vi "Order Controls.vi"(10 "TermBnds[]":T1[](array[typedef]), 11 "Controls in":refnum<vi>[](array[refnum])) -> (1 "sorted array":cluster{"Rectangle":T1, refnum<vi>}[](array[cluster]), 2 "Control locations":T1[](array[typedef]), 3 "Controls out":refnum<vi>[](array[refnum]))   [LabVIEW 2014]
uses:
  <vilib>/Utility/miscctls.llb/LVRectTypeDef.ctl
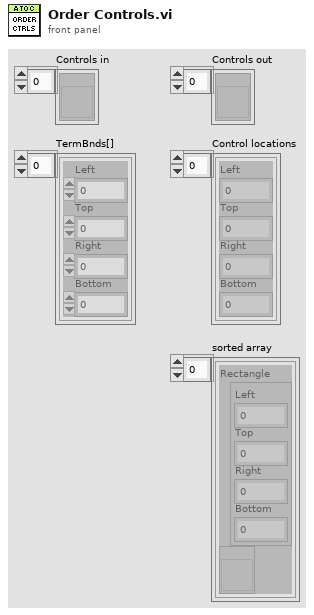
[diagram p1: front panel]
types:
  T1 = typedef "LVRectTypeDef.ctl" = cluster{"Left":i16, "Top":i16, "Right":i16, "Bottom":i16}
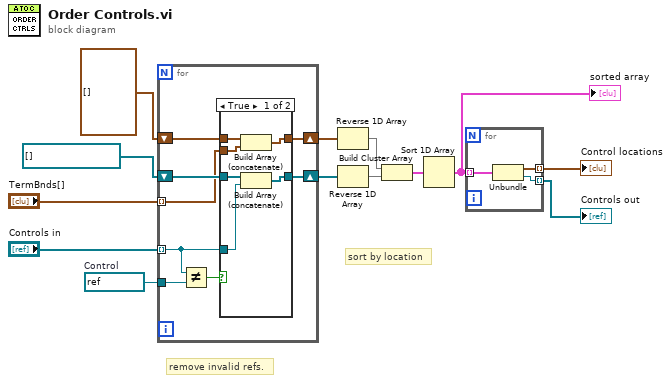
[diagram p0: block diagram]
diagram:
  w13 = refnum<vi> refnum  # Control
  # "sort by location"
  # "remove invalid refs."
  n1 = for {
    tunnel: w13 -> [w17]
    shift-right: [w20] -> w7
    shift-left: refnum<vi>[] [] ("Controls in") -> [w21]
    shift-right: [w18] -> w8
    shift-left: T1[] [] ("TermBnds[]") -> [w19]
    tunnel: "Controls in" -> [w15] mode=indexing
    tunnel: "TermBnds[]" -> [w14] mode=indexing
    n2 = Not Equal?(x=w15, y=w17) -> (x != y?=w16:bool)
    n3 = case shown="True" w16 {
      tunnel: w21 -> [w27 w29]
      tunnel: [w25 w29] -> w20
      tunnel: w19 -> [w26 w28]
      tunnel: [w24 w28] -> w18
      tunnel: w15 -> [w23 _]
      tunnel: w14 -> [w22 _]
      frame True {
        n4 = Build Array (concatenate)(w26, w22) -> (w24:T1[])
        n5 = Build Array (concatenate)(w27, w23) -> (w25:refnum<vi>[])
      }
      frame False {
      }
    }
  }
  n6 = Reverse 1D Array(array=w8) -> (reversed array=w4:T1[])
  n7 = Reverse 1D Array(array=w7) -> (reversed array=w3:refnum<vi>[])
  n8 = Build Cluster Array(w4, w3) -> (w2:cluster{"Rectangle":T1, refnum<vi>}[])
  n9 = Sort 1D Array(array=w2) -> (sorted array=w1:cluster{"Rectangle":T1, refnum<vi>}[])
  "sorted array" <- w1
  n10 = for {
    tunnel: w1 -> [w32] mode=indexing
    tunnel: [w31] -> w6 mode=indexing
    tunnel: [w30] -> w5 mode=indexing
    n11 = Unbundle(w32) -> ("Rectangle"=w30:T1, w31:refnum<vi>)
  }
  "Control locations" <- w5
  "Controls out" <- w6
